vi "map bundle or unbundle to subvi.vi"(8 "error in (no error)":errorcluster, 9 "Controls/Indicators":refnum<vi>[](array[refnum]), 10 "Terms[]":refnum<vi>[](array[refnum]), 11 "SubVI in":refnum<vi>) -> (0 "error out":errorcluster)   [LabVIEW 2013]
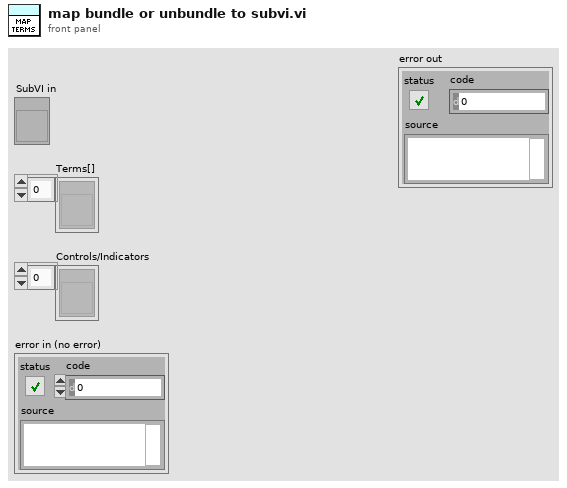
[diagram p1: front panel]
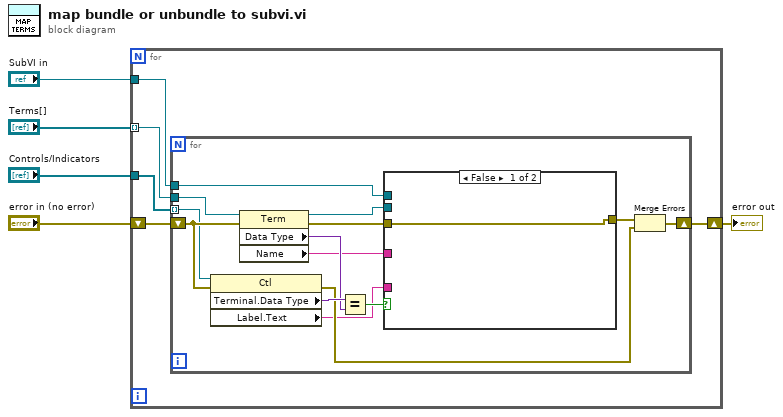
[diagram p0: block diagram]
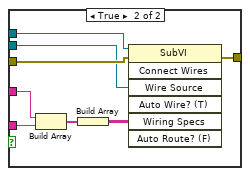
[diagram p2: hidden frame]
diagram:
  n1 = for {
    tunnel: "Terms[]" -> [w10] mode=indexing
    tunnel: "Controls/Indicators" -> [w9]
    shift-right: [w7] -> w1
    shift-left: "error in (no error)" -> [w8]
    tunnel: "SubVI in" -> [w6]
    n2 = for {
      tunnel: w10 -> [w24]
      tunnel: w9 -> [w15] mode=indexing
      shift-right: [w16] -> w7
      shift-left: w8 -> [w20]
      tunnel: w6 -> [w14]
      n3 = property class="Ctl"(reference=w15, error in=w20) -> (error out=w17:errorcluster, "Terminal.Data Type"=w23:variant, "Label.Text"=w11:string)  [unwired: 1 out]
      n4 = property class="Term"(reference=w24, error in=w20) -> (reference out=w21:refnum<vi>, error out=w19:errorcluster, "Data Type"=w22:variant, "Name"=w12:string)
      n5 = Equal?(x=w23, y=w22) -> (x = y?=w13:bool)
      n6 = case shown="False" w13 {
        tunnel: w21 -> [_ w30]
        tunnel: w19 -> [w25 w33]
        tunnel: [w25 w32] -> w18
        tunnel: w14 -> [_ w31]
        tunnel: w12 -> [_ w29]
        tunnel: w11 -> [_ w28]
        frame False {
        }
        frame True {
          n7 = Build Array(w29, w28) -> (w27:string[])
          n8 = Build Array(w27) -> (w26:string[][])
          n9 = invoke class="SubVI" method="Connect Wires"(reference=w31, error in=w33, "Wire Source"=w30, "Wiring Specs"=w26) -> (error out=w32:errorcluster)  [unwired: 3 in, 6 out]
        }
      }
      n10 = Merge Errors(w18, w17) -> (w16:errorcluster)
    }
  }
  "error out" <- w1
